vi "ulozSoubor.vi"(8 "vstupniError":errorcluster, 11 "vstupniNotifier":refnum<notifier>) -> (0 "vystupniError":errorcluster, 2 "vystupniString":string[](array[string]), 3 "vystupWaveforma":waveform(dbl)[](array[waveform]))   [LabVIEW 2018]
panel:
  # "Vstupy:"
  # "Vystupy:"
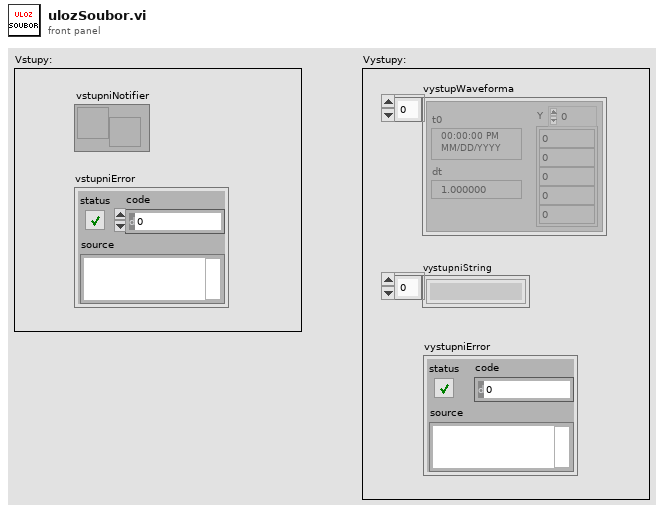
[diagram p1: front panel]
types:
  T1 = enum16{"open", "open or create", "create or replace", "create", "open (read-only)"}
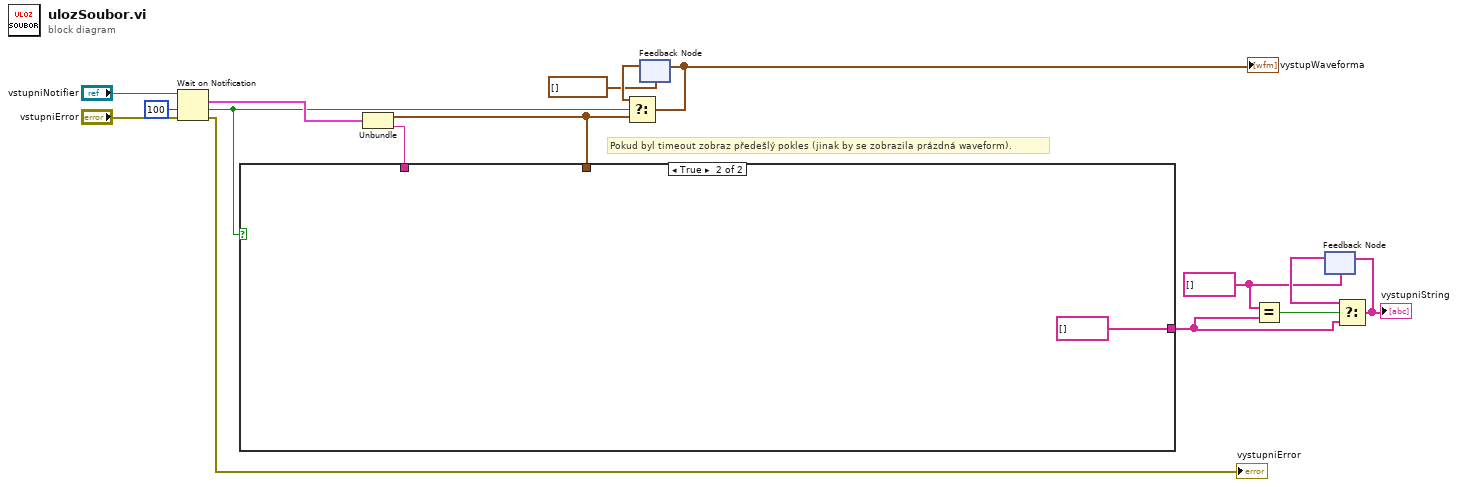
[diagram p0: block diagram]
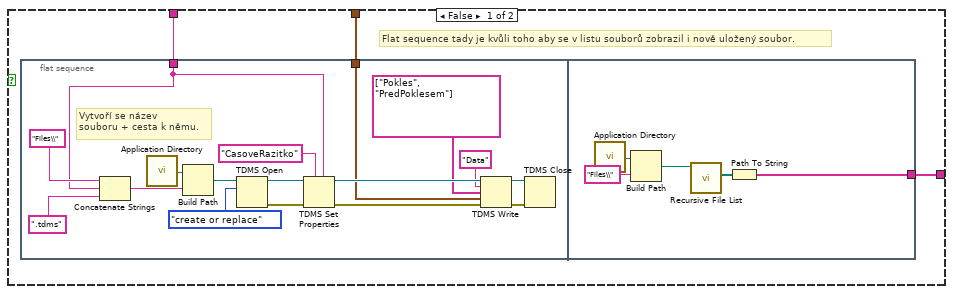
[diagram p2: hidden frame]
diagram:
  w1 = string[] [] ("x")
  # "Pokud byl timeout zobraz předešlý pokles (jinak by se zobrazila prázdná waveform)."
  n1 = Wait on Notification(notifier="vstupniNotifier", timeout in ms (-1)=100, error in (no error)="vstupniError") -> (notification=w13:cluster{waveform(dbl)[], string}, timed out?=w9:bool, error out=→"vystupniError":errorcluster)  [unwired: 1 in, 1 out]
  n2 = Unbundle(w13) -> (w15:waveform(dbl)[], w16:string)
  n3 = case shown="True" w9 {
    tunnel: w15 -> [w19 _]
    tunnel: w16 -> [w18 _]
    tunnel: [w17 string[] [] ("Item Names")] -> w6
    frame False {
      # "Flat sequence tady je kvůli toho aby se v listu souborů zobrazil i nově uložený soubor."
      n4 = flat-sequence {
        tunnel: w19 -> [w24]
        tunnel: w18 -> [w21]
        tunnel: [w37] -> w17
        frame #0 {
          # "Vytvoří se název \nsouboru + cesta k němu."
          n5 = Concatenate Strings("Files\\" ("name or relative path"), w21, ".tdms" ("name or relative path")) -> (w20:string)
          n6 = call <vilib>:"Application Directory.vi"() -> ("Application Directory"=w29:path)
          n7 = Build Path(base path=w29, name or relative path=w20) -> (appended path=w30:path)
          n8 = TDMS Open(10:T1."create or replace" ("operation (0:open)"), 11:w30) -> (0:w32:errorcluster, 3:w31:refnum<k34>)  [unwired: 5 in]
          n9 = TDMS Set Properties(5:w21, 7:"CasoveRazitko" ("element"), 8:w32, 11:w31) -> (0:w36:errorcluster, 3:w35:refnum<k34>)  [unwired: 2 in, 2 out]
          n10 = TDMS Write(0:w35, 5:"Data" ("group name in (Untitled)"), 7:string[] ["Pokles", "PredPoklesem"], 9:w24, 11:w36) -> (4:w33:refnum<k34>, 15:w34:errorcluster)  [unwired: 1 in, 2 out]
          n11 = TDMS Close(8:w34, 11:w33) -> ()  [unwired: 2 out]
        }
        frame #1 {
          n12 = call <vilib>:"Application Directory.vi"() -> ("Application Directory"=w41:path)
          n13 = Build Path(base path=w41, name or relative path="Files\\") -> (appended path=w40:path)
          n14 = call <vilib>:"Recursive File List.vi"("Folder Path"=w40) -> ("All Files in Dir"=w39:path[])  [unwired: 6 in, 4 out]
          n15 = Path To String(path=w39) -> (string=w37:string[])
        }
      }
    }
    frame True {
    }
  }
  n16 = feedback #1(waveform(dbl)[] [] ("s? t:f")) -> (w3:waveform(dbl)[])
  n17 = Select(t=w3, s=w9, f=w15) -> (s? t:f=w4:waveform(dbl)[])
  "vystupWaveforma" <- w4
  n18 = feedback-in #1(w4) -> ()
  n19 = Equal?(x=w1, y=w6) -> (x = y?=w8:bool)
  n20 = feedback #2(w1) -> (w7:string[])
  n21 = Select(t=w7, s=w8, f=w6) -> (s? t:f=w5:string[])
  "vystupniString" <- w5
  n22 = feedback-in #2(w5) -> ()
